vi "newporttesting.vi"() -> ()   [LabVIEW 2014]
panel:
  out "TimeoutFlag 3":bool
  out "Response 3":string
  out "Response 2":string
  out "TimeoutFlag 2":bool
  out "error out":errorcluster
  out "Response":string
  out "TimeoutFlag":bool
  in  "Visa Session":refnum<visa-resource-name>
  in  "Controller #":string
  in  "error in (no error)":errorcluster
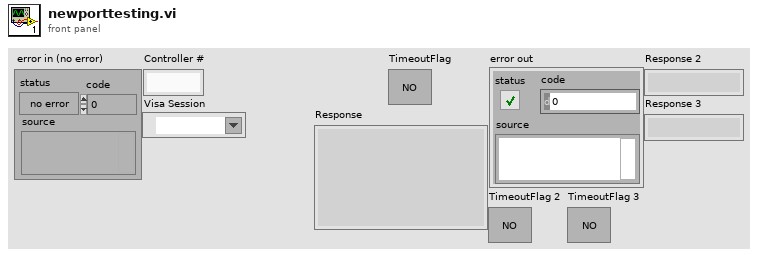
[diagram p1: front panel]
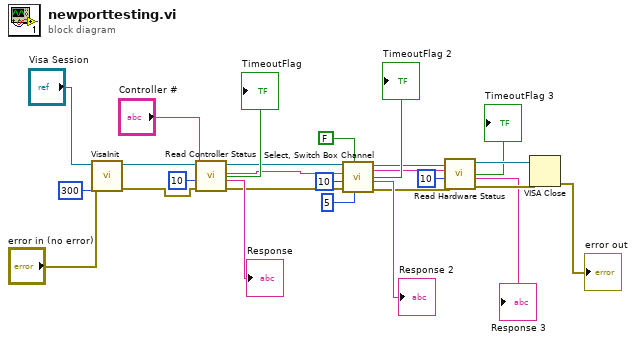
[diagram p0: block diagram]
diagram:
  n1 = call <userlib>:"VisaInit.vi"("error in (no error)"="error in (no error)", "Timeout (ms)"=u32 300, "Visa Session"="Visa Session") -> ("error out"=w21:errorcluster, "Visa Handle"=w23:refnum<visa-resource-name>)  [unwired: 4 in]
  n2 = call <userlib>:"Read Controller Status.vi"("error in (no error)"=w21, "Delay (ms)"=u32 10, "Controller #"="Controller #", "VISA Handle"=w23) -> ("error out"=w15:errorcluster, "Response"=→"Response":string, "Dup Controller #"=w14:string, "Dup VISA Handle"=w16:refnum<visa-resource-name>, "TimeoutFlag"=→"TimeoutFlag":bool)  [unwired: 1 in]
  n3 = call <userlib>:"Select, Switch Box Channel.vi"("Value"=5, "Query?"=FALSE, "error in (no error)"=w15, "Delay (ms)"=u32 10, "Controller #"=w14, "VISA Handle"=w16) -> ("error out"=w8:errorcluster, "Response"=→"Response 2":string, "Dup Controller #"=w7:string, "Dup VISA Handle"=w6:refnum<visa-resource-name>, "TimeoutFlag"=→"TimeoutFlag 2":bool)
  n4 = call <userlib>:"Read Hardware Status.vi"("error in (no error)"=w8, "Delay (ms)"=u32 10, "Controller #"=w7, "VISA Handle"=w6) -> ("error out"=w4:errorcluster, "Response"=→"Response 3":string, "Dup VISA Handle"=w2:refnum<visa-resource-name>, "TimeoutFlag"=→"TimeoutFlag 3":bool)  [unwired: 1 in, 1 out]
  n5 = VISA Close(VISA resource name=w2, error in (no error)=w4) -> (error out=→"error out":errorcluster)
